vi "CapturePacket.vi"(0 "Buffer":string) -> (1 "Buffer":string, 2 "Packet":string, 3 "Packet Located":bool, 4 "Packet Size":i32)   [LabVIEW 2015, in "navX Library v3.lvlib" / "navX - SERIAL.lvclass"]
uses:
  navX - SERIAL.lvclass
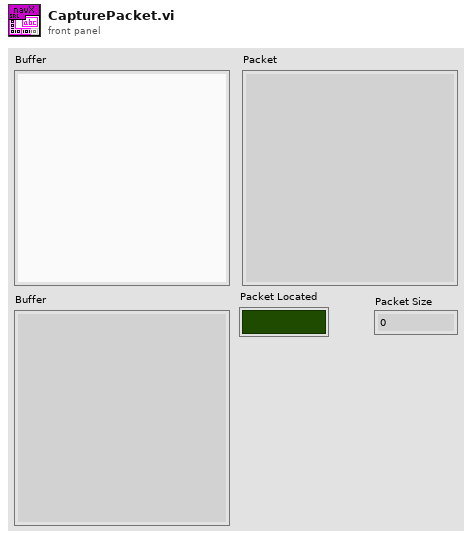
[diagram p1: front panel]
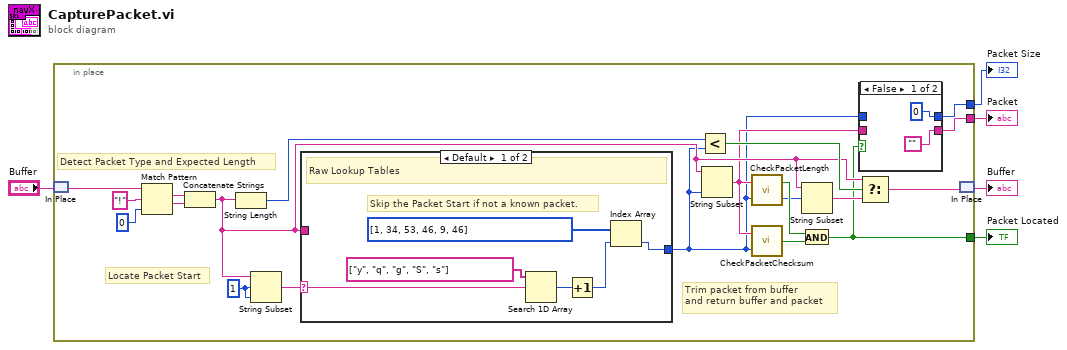
[diagram p0: block diagram]
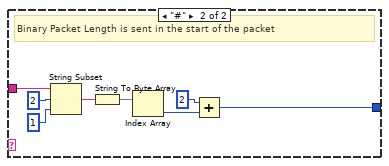
[diagram p2: hidden frame]
diagram:
  n1 = in-place {
    in-place-border: [w14] -> w3
    in-place-border: [w13] -> w2
    in-place-border: [w11] -> w1
    w25 = 1 ("length (rest)")
    # "Locate Packet Start"
    # "Trim packet from buffer\nand return buffer and packet"
    # "Detect Packet Type and Expected Length"
    n2 = in-place-match #1("Buffer") -> (w15:string)
    n3 = Match Pattern(string=w15, regular expression="!" ("Packet Start Char"), offset (0)=0 ("offset past match")) -> (match substring=w23:string, after substring=w22:string)  [unwired: 2 out]
    n4 = Concatenate Strings(w23, w22) -> (w17:string)
    n5 = String Length(string=w17) -> (length=w19:i32)
    n6 = String Subset(string=w17, offset (0)=w25, length (rest)=w25) -> (substring=w24:string)
    n7 = case shown="Default" w24 {
      selector: w24 -> [w27 _]
      tunnel: [w28 w35] -> w8
      tunnel: w17 -> [_ w33]
      frame Default {
        # "Skip the Packet Start if not a known packet."
        # "Raw Lookup Tables"
        n8 = Search 1D Array(1D array=string[] ["y", "q", "g", "S", "s"], element=w27) -> (index of element=w29:i32)  [unwired: 1 in]
        n9 = Increment(x=w29) -> (x+1=w26:i32)
        n10 = Index Array(array=i32[] [1, 34, 53, 46, 9, 46], index=w26) -> (element=w28:i32)
      }
      frame "#" {
        # "Binary Packet Length is sent in the start of the packet"
        n11 = String Subset(string=w33, offset (0)=2, length (rest)=1 ("length (rest)")) -> (substring=w34:string)
        n12 = String To Byte Array(string=w34) -> (unsigned byte array=w37:u8[])
        n13 = Index Array(array=w37) -> (element=w38:u8)  [unwired: 1 in]
        n14 = Add(x=u8 2 ("y"), y=w38) -> (x+y=w35:u8)
      }
    }
    n15 = Less?(x=w19, y=w8) -> (x < y?=w18:bool)
    n16 = String Subset(string=w17, length (rest)=w8) -> (substring=w9:string)  [unwired: 1 in]
    n17 = call "CheckPacketLength.vi"("Expected Packet Length"=w8, "Buffer"=w9) -> ("Packet Termination Offset"=w6:i32, "Packet Valid"=w7:bool)
    n18 = call "CheckPacketChecksum.vi"("Expected Packet Length"=w8, "Buffer"=w9) -> ("Packet Valid"=w10:bool)
    n19 = String Subset(string=w17, offset (0)=w6) -> (substring=w16:string)  [unwired: 1 in]
    n20 = And(x=w7, y=w10) -> (x .and. y?=w11:bool)
    n21 = case shown="False" w11 {
      tunnel: ["" w43] -> w13
      tunnel: w9 -> [_ w43]
      tunnel: [0 w42] -> w14
      tunnel: w8 -> [_ w42]
      frame False {
      }
      frame True {
      }
    }
    n22 = Select(t=w17, s=w18, f=w16) -> (s? t:f=w12:string)
    n23 = in-place-match #1(w12) -> (→"Buffer":string)
  }
  "Packet" <- w2
  "Packet Located" <- w1
  "Packet Size" <- w3
